vi "roi2xy.vi"(5 "ROI":i32[](array[numeric])) -> (1 "xy":i32[](array[numeric]))   [LabVIEW 2011]
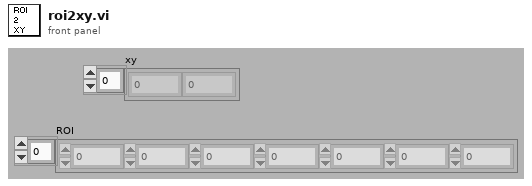
[diagram p1: front panel]
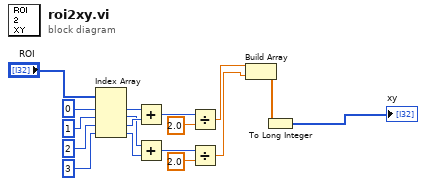
[diagram p0: block diagram]
diagram:
  n1 = Index Array(array="ROI", index #1=0 ("index"), index #2=1 ("index"), index #3=2 ("index"), index #4=3 ("index")) -> (element #1=w9:i32, element #2=w5:i32, element #3=w8:i32, element #4=w4:i32)
  n2 = Add(x=w9, y=w8) -> (x+y=w10:i32)
  n3 = Add(x=w5, y=w4) -> (x+y=w6:i32)
  n4 = Divide(x=w10, y=2.0) -> (x/y=w2:dbl)
  n5 = Divide(x=w6, y=2.0) -> (x/y=w1:dbl)
  n6 = Build Array(w2, w1) -> (w12:dbl[])
  n7 = To Long Integer(number=w12) -> (32bit integer=→"xy":i32[])
